vi "call to save.vi"(8 "error in":errorcluster, 11 "DAQCascade512II":refnum<class "DAQCascade512II.lvclass">) -> (0 "error out":errorcluster, 3 "DAQCascade512II out":refnum<class "DAQCascade512II.lvclass">)   [LabVIEW 2012, in "DAQCascade512II.lvclass"]
uses:
  DAQCascade512II.lvclass
  DAQCascade512II.lvclass/DAQCascade512II.ctl
panel:
  in  "ref path":path=path "C:/DATA/Programming/Giorgio/DAQCascade512II/Get images from queue.vi"
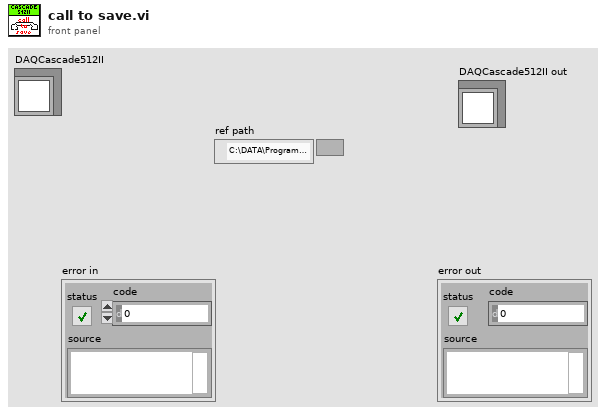
[diagram p1: front panel]
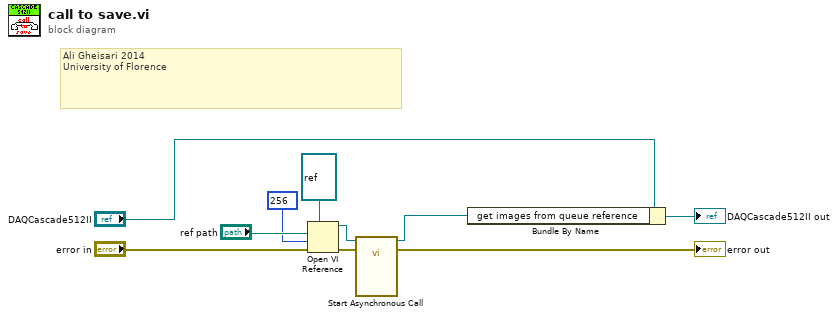
[diagram p0: block diagram]
diagram:
  # "Ali Gheisari 2014\nUniversity of Florence"
  n1 = Open VI Reference(type specifier VI Refnum (for type only)=refnum<vi> refnum, vi path="ref path", options=256, error in (no error)="error in") -> (vi reference=w6:refnum<vi>, error out=w5:errorcluster)  [unwired: 2 in]
  n2 = call-by-ref "Start Asynchronous Call"(reference=w6, error in=w5) -> (reference out=w1:refnum<vi>, error out=→"error out":errorcluster)  [unwired: 11 in, 1 out]
  n3 = Bundle By Name(cluster="DAQCascade512II", "get images from queue reference"=w1) -> (→"DAQCascade512II out":refnum<class "DAQCascade512II.lvclass">)
